vi "Dialog.Simple Text Info.vi"(9 "Text In":string="Info XXX", 11 "Title":string="Info") -> ()   [LabVIEW 2018]
uses:
  <vilib>/KATE/Queues/Queue Utils.lvlib
  <vilib>/KATE/Controls/Controls.lvlib
panel:
  in  "Main Tab":enum32{"Data", "Setup"}(tab)
  out "Text":string
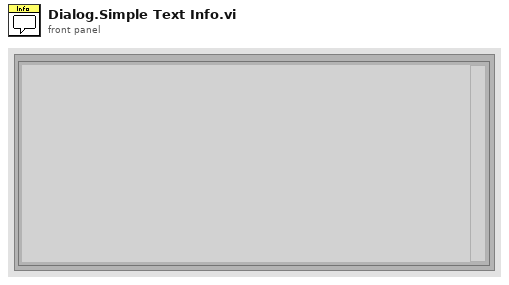
[diagram p1: front panel]
types:
  T1 = enum32{"Invalid", "Standard", "Closed", "Hidden", "Minimized", "Maximized"}
  T2 = enum16{"Top Left", "Bottom Right", "Top Right", "Bottom Left"}
  T3 = enum16{"Top Left", "Top Right", "Bottom Left", "Bottom Right"}
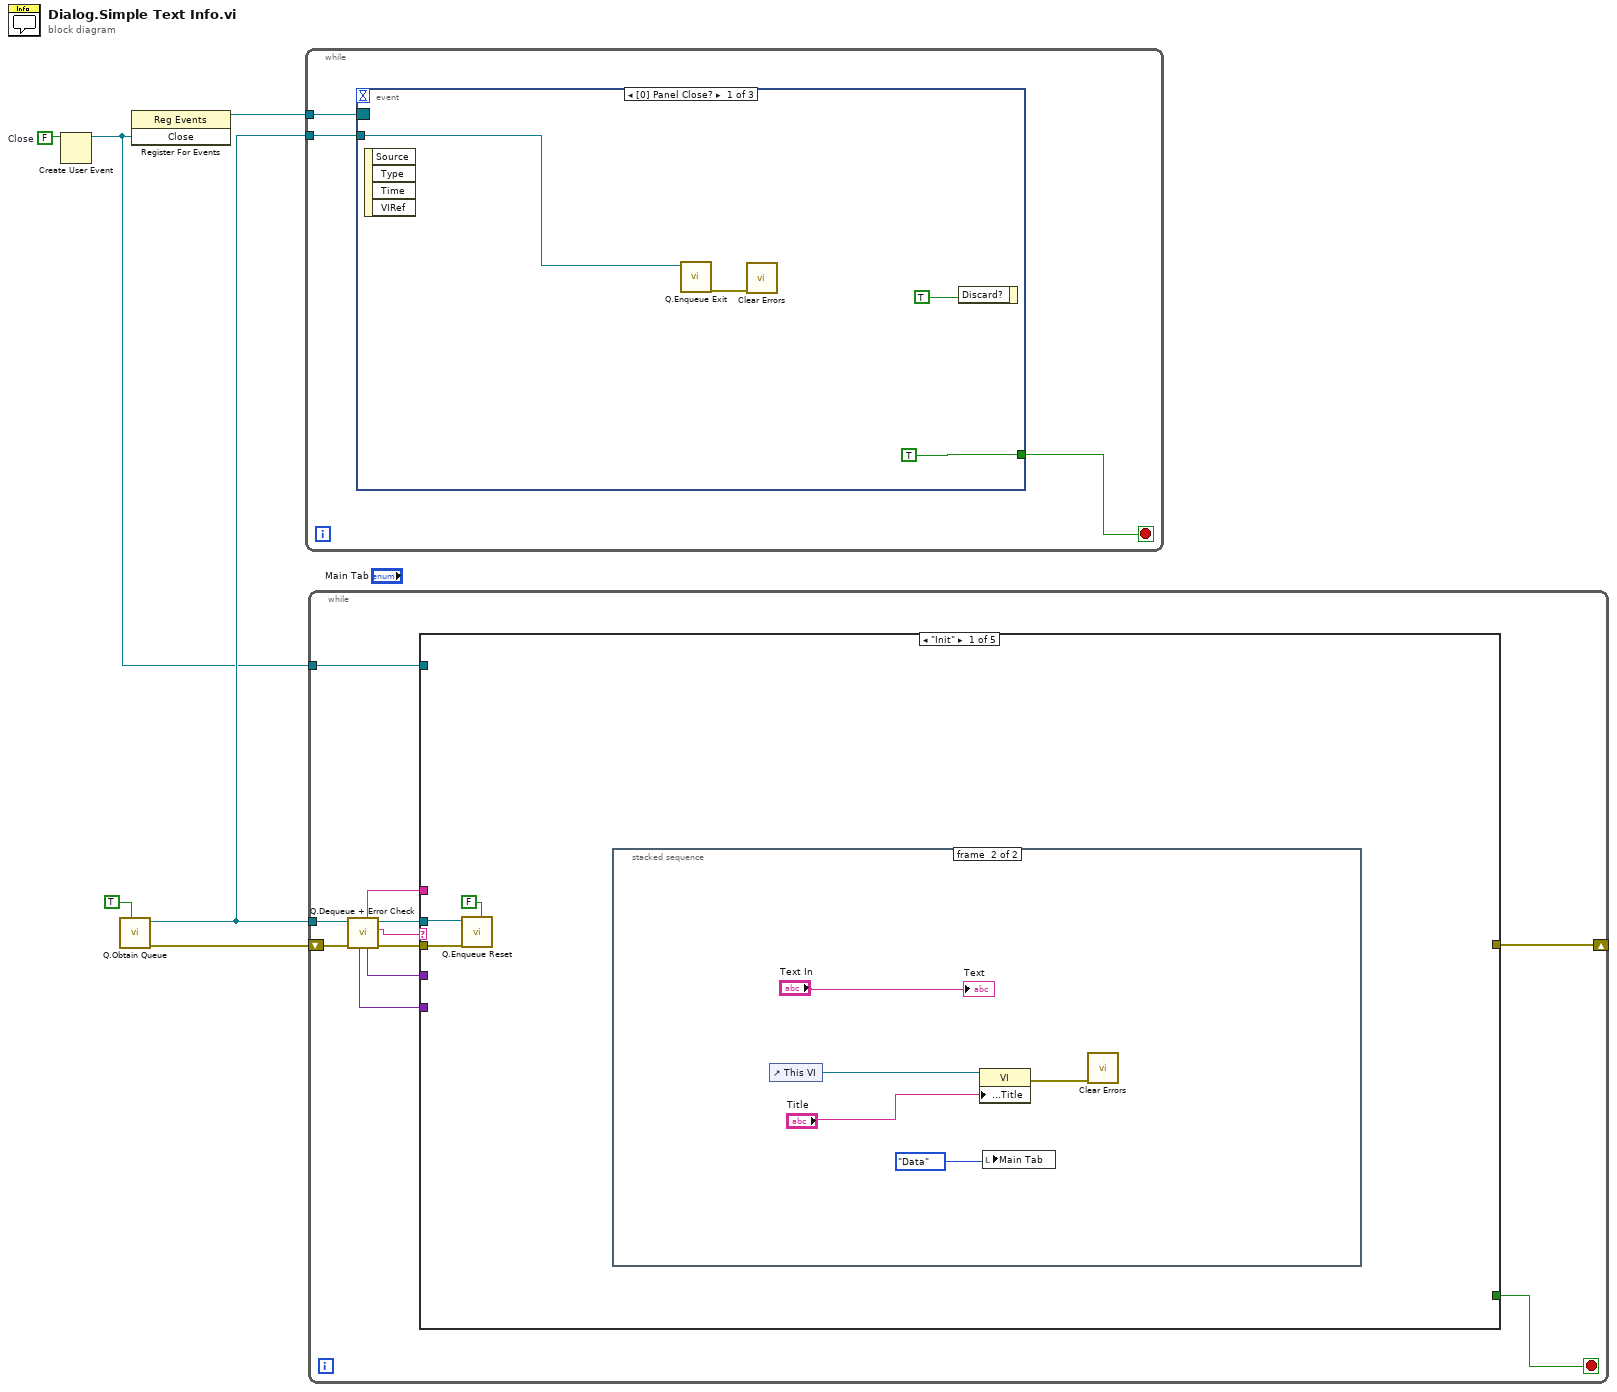
[diagram p0: block diagram]
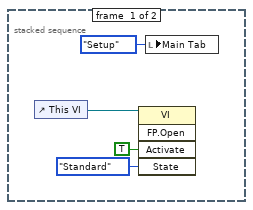
[diagram p2: hidden frame]
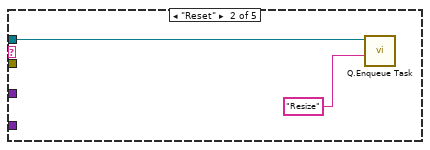
[diagram p3: hidden frame]
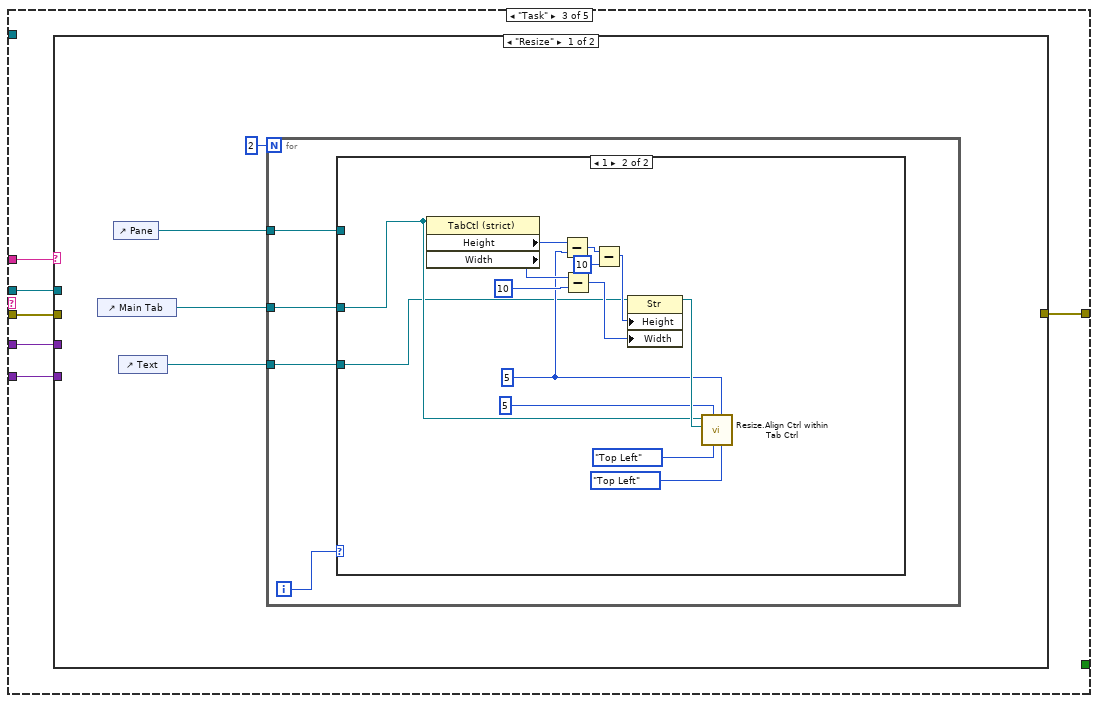
[diagram p4: hidden frame]
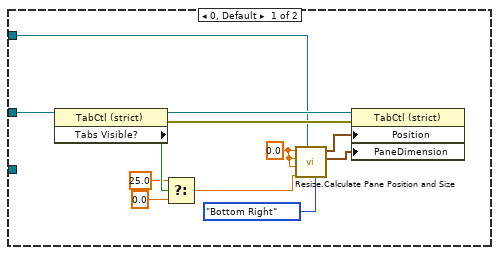
[diagram p5: hidden frame]
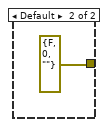
[diagram p6: hidden frame]
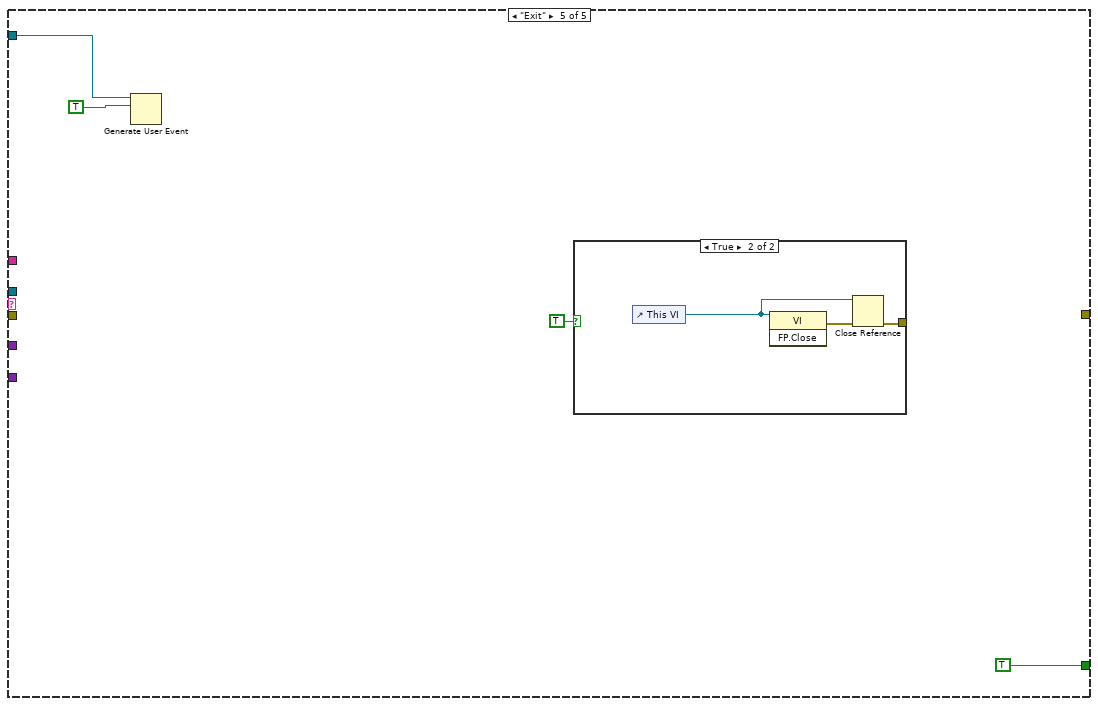
[diagram p8: hidden frame]
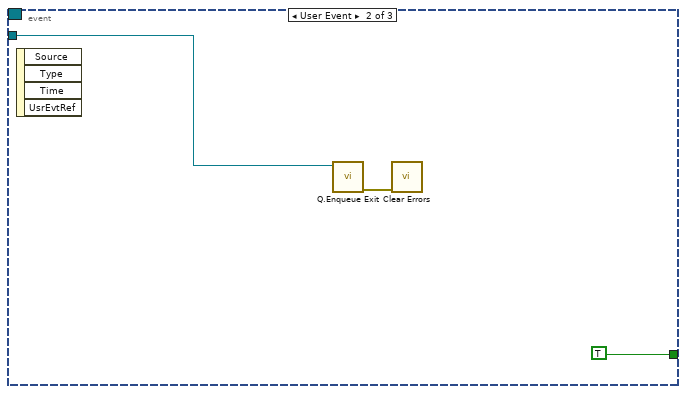
[diagram p10: hidden frame]
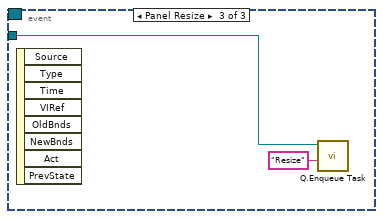
[diagram p11: hidden frame]
diagram:
  w6 = FALSE  # Close
  n1 = Create User Event(user event datatype=w6) -> (user event=w1:refnum<user-event>)  [unwired: 1 in, 1 out]
  n2 = call <vilib>:"Q.Obtain Queue.vi"("Enqueue Init"=TRUE) -> ("error out"=w3:errorcluster, "Q Out"=w2:refnum<queue>)  [unwired: 8 in, 1 out]
  n3 = register-events(w1) -> (reference out=w5:refnum<event-registration>)  [unwired: 2 in, 1 out]
  n4 = while {
    tunnel: w5 -> [w9]
    tunnel: w2 -> [w8]
    stop <- w7 stop-if-true
    n5 = event shown="[0] Panel Close?" {
      selector: w9 -> [_ _ _]
      dyn-events: _ -> [_ _ _]
      timeout: _ -> [_ _ _]
      tunnel: w8 -> [w12 w15 w18]
      tunnel: [TRUE TRUE _] -> w7
      event Panel Close? {
        n6 = event-data() -> ()  [unwired: 1 in, 4 out]
        n7 = call <vilib>:"Q.Enqueue Exit.vi"("Q In"=w12) -> ("error out"=w11:errorcluster)  [unwired: 9 in, 1 out]
        n8 = call <vilib>:"Clear Errors.vi"("error in (no error)"=w11) -> ()  [unwired: 5 in, 2 out]
        n9 = event-data("Discard?"=TRUE) -> ()  [unwired: 1 in, 1 out]
      }
      event User Event {
        n10 = event-data() -> ()  [unwired: 1 in, 4 out]
        n11 = call <vilib>:"Q.Enqueue Exit.vi"("Q In"=w15) -> ("error out"=w14:errorcluster)  [unwired: 9 in, 1 out]
        n12 = call <vilib>:"Clear Errors.vi"("error in (no error)"=w14) -> ()  [unwired: 5 in, 2 out]
      }
      event Panel Resize {
        n13 = event-data() -> ()  [unwired: 1 in, 8 out]
        n14 = call <vilib>:"Q.Enqueue Task.vi"("Task Name"="Resize", "Q In"=w18) -> ()  [unwired: 8 in, 2 out]
      }
    }
  }
  n15 = while {
    shift-right: [w21] -> _
    shift-left: w3 -> [w26]
    tunnel: w2 -> [w24]
    tunnel: w1 -> [w19]
    stop <- w20 stop-if-true
    n16 = call <vilib>:"Q.Dequeue + Error Check.vi"("Error In"=w26, "Q In"=w24) -> ("error out"=w27:errorcluster, "Cmd"=w29:string, "Q Out"=w28:refnum<queue>, "Data1"=w23:variant, "Sub"=w25:string, "Data2"=w22:variant)  [unwired: 4 in]
    n17 = case shown="\"Init\"" w29 {
      tunnel: w28 -> [w32 w42 w48 _ _]
      tunnel: w27 -> [w31 _ w47 _ _]
      tunnel: w25 -> [_ _ w49 _ _]
      tunnel: w23 -> [_ _ w46 _ _]
      tunnel: w22 -> [_ _ w45 _ _]
      tunnel: [_ _ w44 _ _] -> w21
      tunnel: [_ _ _ _ TRUE] -> w20
      tunnel: w19 -> [_ _ _ _ w87]
      frame "Init" {
        n18 = call <vilib>:"Q.Enqueue Reset.vi"("Top of Q(T)"=FALSE, "Error In"=w31, "Q In"=w32) -> ()  [unwired: 7 in, 2 out]
        n19 = stacked-sequence {
          frame #0 {
            n20 = control-ref of="This VI"() -> (w36:refnum<vi>)
            n21 = invoke class="VI" method="FP.Open"(reference=w36, "Activate"=TRUE ("Activate?"), "State"=T1."Standard") -> ()  [unwired: 2 in, 5 out]
            n22 = local write "Main Tab"(enum32{"Data", "Setup"}."Setup" ("Main Tab")) -> ()
          }
          frame #1 {
            n23 = control-ref of="This VI"() -> (w41:refnum<vi>)
            n24 = property class="VI"(reference=w41, "Front Panel.Title"="Title") -> (error out=w40:errorcluster)  [unwired: 1 in, 1 out]
            n25 = local write "Main Tab"(enum32{"Data", "Setup"}."Data" ("Main Tab")) -> ()
            n26 = call <vilib>:"Clear Errors.vi"("error in (no error)"=w40) -> ()  [unwired: 5 in, 2 out]
            "Text" <- "Text In"
          }
        }
      }
      frame "Reset" {
        n27 = call <vilib>:"Q.Enqueue Task.vi"("Task Name"="Resize", "Q In"=w42) -> ()  [unwired: 8 in, 2 out]
      }
      frame "Task" {
        n28 = case shown="\"Resize\"" w49 {
          tunnel: w48 -> [_ _]
          tunnel: w47 -> [_ _]
          tunnel: w46 -> [_ _]
          tunnel: w45 -> [_ _]
          tunnel: [_ errorcluster {"status"=FALSE, "code"=0, "source"=""} ("error constant")] -> w44
          frame "Resize" {
            n29 = control-ref of="Main Tab"() -> (w53:refnum<vi>)
            n30 = control-ref of="Pane"() -> (w51:refnum<vi>)
            n31 = control-ref of="Text"() -> (w52:refnum<vi>)
            n32 = for {
              N: 2 -> [_]
              tunnel: w53 -> [w56]
              tunnel: w52 -> [w55]
              tunnel: w51 -> [w54]
              i -> [w57]
              n33 = case shown="1" w57 {
                tunnel: w56 -> [w59 w71]
                tunnel: w55 -> [_ w70]
                tunnel: w54 -> [w58 _]
                frame 0, Default {
                  w62 = 0.0 ("X Origin")
                  n34 = property class="TabCtl (strict)"(reference=w59) -> (reference out=w69:refnum<vi>, error out=w65:errorcluster, "Tabs Visible?"=w68:bool)  [unwired: 1 in]
                  n35 = Select(t=25.0, s=w68, f=0.0) -> (s? t:f=w61:dbl)
                  n36 = call <vilib>:"Resize.Calculate Pane Position and Size.vi"("Origin for X,Y Max (Top Left)"=T2."Bottom Right", "Pane in"=w58, "Y Max"=w61, "X Max"=w62, "Y Origin"=w62, "X Origin"=w62) -> ("Size"=w63:cluster{u32, u32}, "Position"=w64:cluster{"X Coordinate":i32, "Y Coordinate":i32})  [unwired: 4 in]
                  n37 = property class="TabCtl (strict)"(reference=w69, error in=w65, "Position"=w64, "PaneDimension"=w63) -> ()  [unwired: 2 out]
                }
                frame 1 {
                  w73 = u32 5 ("y")
                  n38 = property class="TabCtl (strict)"(reference=w71) -> ("Height"=w81:u32, "Width"=w80:u32)  [unwired: 1 in, 2 out]
                  n39 = Subtract(x=w81, y=w73) -> (x-y=w77:u32)
                  n40 = Subtract(x=w80, y=u32 10) -> (x-y=w78:u32)
                  n41 = Subtract(x=w77, y=u32 10) -> (x-y=w75:u32)
                  n42 = property class="Str"(reference=w70, "Height"=w75, "Width"=w78) -> (reference out=w74:refnum<vi>)  [unwired: 1 in, 1 out]
                  n43 = call <vilib>:"Resize.Align Ctrl within Tab Ctrl.vi"("Child Ref Pos"=T3."Top Left", "dY"=w73, "Parent Ref Pos"=T3."Top Left", "dX"=u32 5 ("y"), "Child Ctrl"=w74, "Parent Tab Ctrl"=w71) -> ()  [unwired: 3 in, 3 out]
                }
              }
            }
          }
          frame Default {
          }
        }
      }
      frame "Error", Default {
        # "Do Nothing (for now)"
      }
      frame "Exit" {
        n44 = Generate User Event(user event=w87, event data cluster=TRUE ("event data")) -> ()  [unwired: 2 in, 2 out]
        n45 = case shown="True" TRUE {
          tunnel: [_ w89] -> _
          frame False {
          }
          frame True {
            n46 = control-ref of="This VI"() -> (w91:refnum<vi>)
            n47 = invoke class="VI" method="FP.Close"(reference=w91) -> (error out=w90:errorcluster)  [unwired: 2 in, 2 out]
            n48 = Close Reference(reference=w91, error in (no error)=w90) -> (error out=w89:errorcluster)
          }
        }
      }
    }
  }
